vi "Tray Data and Total.vi"(9 "Data in":string[](array[string]), 10 "ROW":u8, 11 "COL":u8) -> (2 "TrayData":bool[](array[boolean]), 3 "Total":i32)   [LabVIEW 2015]
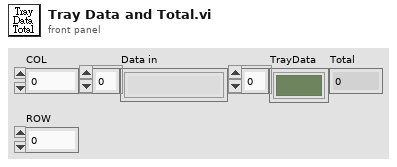
[diagram p1: front panel]
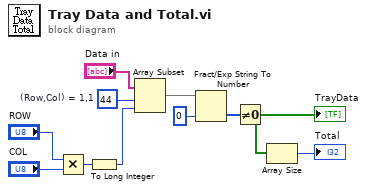
[diagram p0: block diagram]
diagram:
  w6 = 44  # (Row,Col) = 1,1
  n1 = Multiply(x="ROW", y="COL") -> (x*y=w10:u8)
  n2 = To Long Integer(number=w10) -> (32bit integer=w1:i32)
  n3 = Array Subset(array="Data in", index=w6, length=w1) -> (w11:string[])
  n4 = Fract/Exp String To Number(string=w11, default (0 dbl)=0 ("default (0 DBL)")) -> (number=w4:i32[])  [unwired: 2 in, 1 out]
  n5 = Not Equal To 0?(x=w4) -> (x != 0?=w2:bool[])
  "TrayData" <- w2
  n6 = Array Size(array=w2) -> (size(s)=→"Total":i32)
